vi "SetParam.vi"(8 "error in (no error)":errorcluster caption="entrée d'erreur (pas d'erreur)", 10 "binarize":cluster{"threshold":dbl, "copy":bool}={"threshold"=0.0, "copy"=TRUE}, 11 "binarize.lvclass":refnum<class "binarize.lvclass">) -> (0 "error out":errorcluster caption="sortie d'erreur", 3 "binarize.lvclass":refnum<class "binarize.lvclass">)   [LabVIEW 2020, in "binarize.lvclass"]
doc: "Set Parameters"
uses:
  binarize.lvclass
  binarize.lvclass/binarize.ctl
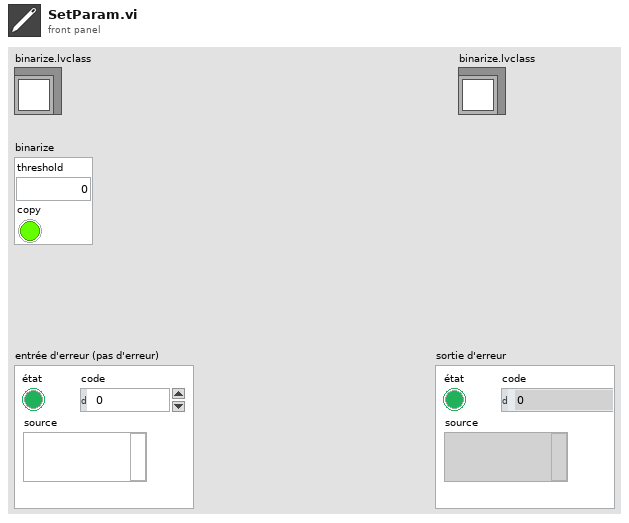
[diagram p1: front panel]
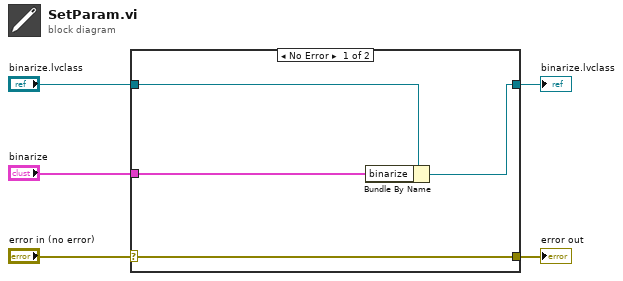
[diagram p0: block diagram]
diagram:
  n1 = case shown="No Error" "error in (no error)" {
    selector: "error in (no error)" -> [w9 w10]
    tunnel: [w9 w10] -> w4
    tunnel: [w7 w11] -> w2
    tunnel: "binarize.lvclass" -> [w8 w11]
    tunnel: "binarize" -> [w6 _]
    frame No Error {
      n2 = Bundle By Name(cluster=w8, "binarize"=w6) -> (w7:refnum<class "binarize.lvclass">)
    }
    frame Error {
    }
  }
  "error out" <- w4
  "binarize.lvclass" <- w2
